vi "Main.vi"() -> ()   [LabVIEW 2016]
doc: "This Continuous Measurement sample project is based on the Queued Message Handler template.\n\nThe Event Handling Loop generates messages based on user interface actions.\n\nThe Message Handling Loop processes messages generated by the Event Handling Loop, or by other messages. There are also Acquisition and Logging message handling loop subVIs, and a chart updating loop."
uses:
  controls/UI State.ctl
  <vilib>/Analysis/baseanly.llb/Mean (DBL).vi
  <vilib>/express/express analysis/Spectral/Block/exnSpectralBlock spectral measurements PSD poly.vi
  <vilib>/express/express analysis/Spectral/Block/exnSpectralBlock spectral measurements PSD DDT.vi
  support/Message Queue/Enqueue Message (Single).vi
  <vilib>/Utility/error.llb/Error Cluster From Error Code.vi
  <vilib>/express/express analysis/Spectral/XNode/ExpressSpectralMeasurementsBlockNode.xnode
  <vilib>/ErrorRing/Error Ring.xnode
  Acquisition/Acquisition.lvlib
  Logging/Logging.lvlib
  Settings/Settings.lvlib
  support/User Event - Stop/User Event - Stop.lvlib
  support/Message Queue/Message Queue.lvlib
  <vilib>/Analysis/NI_AALBase.lvlib
panel:
  out "Y (V)":dbl format="%#_3f"
  out "X (V)":dbl format="%#_3f"
  out "Sum (V)":dbl format="%#_3f"
  out "XY Graph":cluster{"Y":dbl[], "Y":dbl[]}[](graph)
  out "Y":dynamicdata(graph)
  in  "Stop_Log":bool
  in  "Log":bool
  in  "Exit":bool
  out "Status":string
  in  "Settings":bool
  in  "Stop_Acquire":bool
  in  "Acquire":bool
  out "X":dynamicdata(graph)
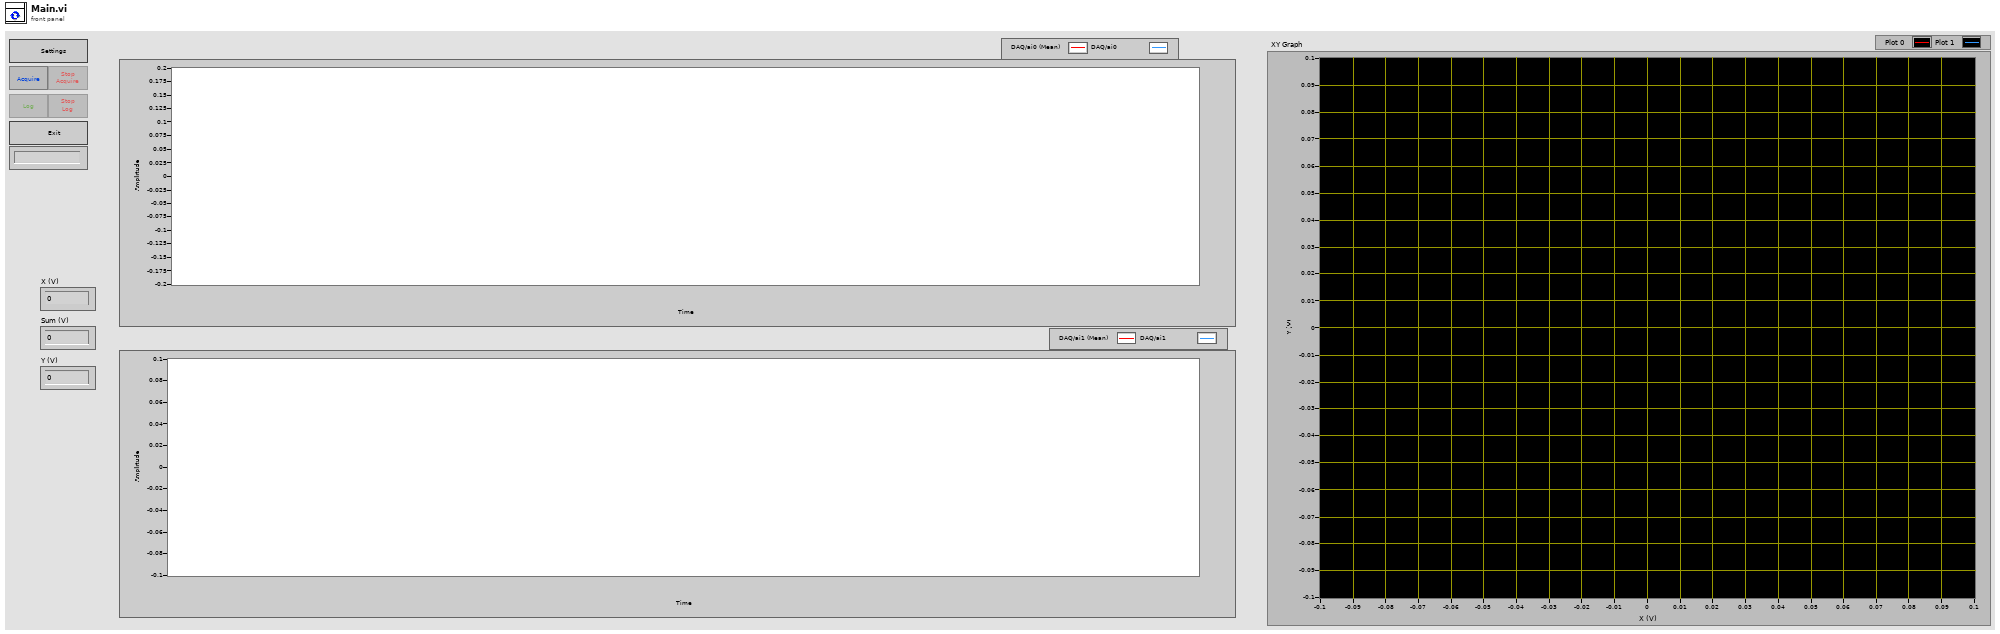
[diagram p1: front panel]
types:
  T1 = typedef "UI State.ctl" = enum16{"Idle", "Acquiring", "Acquiring Stopped", "Logging", "Logging Stopped"}
  T2 = cluster{"Acquire Ref":refnum<vi>, "Log Ref":refnum<vi>, "Stop_Acquire Ref":refnum<vi>, "Settings Ref":refnum<vi>, "Status Ref":refnum<vi>, "Exit Ref":refnum<vi>, "Stop_Log Ref":refnum<vi>}
  T3 = cluster{"Hardware Configuration":cluster{"DAQmx Channel":tag, "Max Input":dbl, "Min Input":dbl, "Sample Rate":dbl, "Channel description":string}, "Logging Configuration":cluster{"Log File Base Path":path, "TDMS File Reference":refnum<k34>, "User":string, "Data description":string}}
  T4 = typedef "Message Queue.lvlib/All Message Queues.ctl" = cluster{"UI":refnum<queue>, "Acquisition":refnum<queue>, "Logging":refnum<queue>}
  T5 = typedef "Settings.lvlib/Settings.ctl" = cluster{"Hardware Configuration":cluster{"DAQmx Channel":tag, "Max Input":dbl, "Min Input":dbl, "Sample Rate":dbl, "Channel description":string}, "Logging Configuration":cluster{"Log File Base Path":path, "TDMS File Reference":refnum<k34>, "User":string, "Data description":string}}
  T6 = cluster{"DAQmx Channel":tag, "Max Input":dbl, "Min Input":dbl, "Sample Rate":dbl, "Channel description":string}
  T7 = cluster{"Log File Base Path":path, "TDMS File Reference":refnum<k34>, "User":string, "Data description":string}
  T8 = cluster{"averaging mode":u16, "weighting mode":u16, "number of averages":u32}
  T9 = cluster{"dB On (F)":bool, "unwrap phase (F)":bool, "convert to degree (F)":bool}
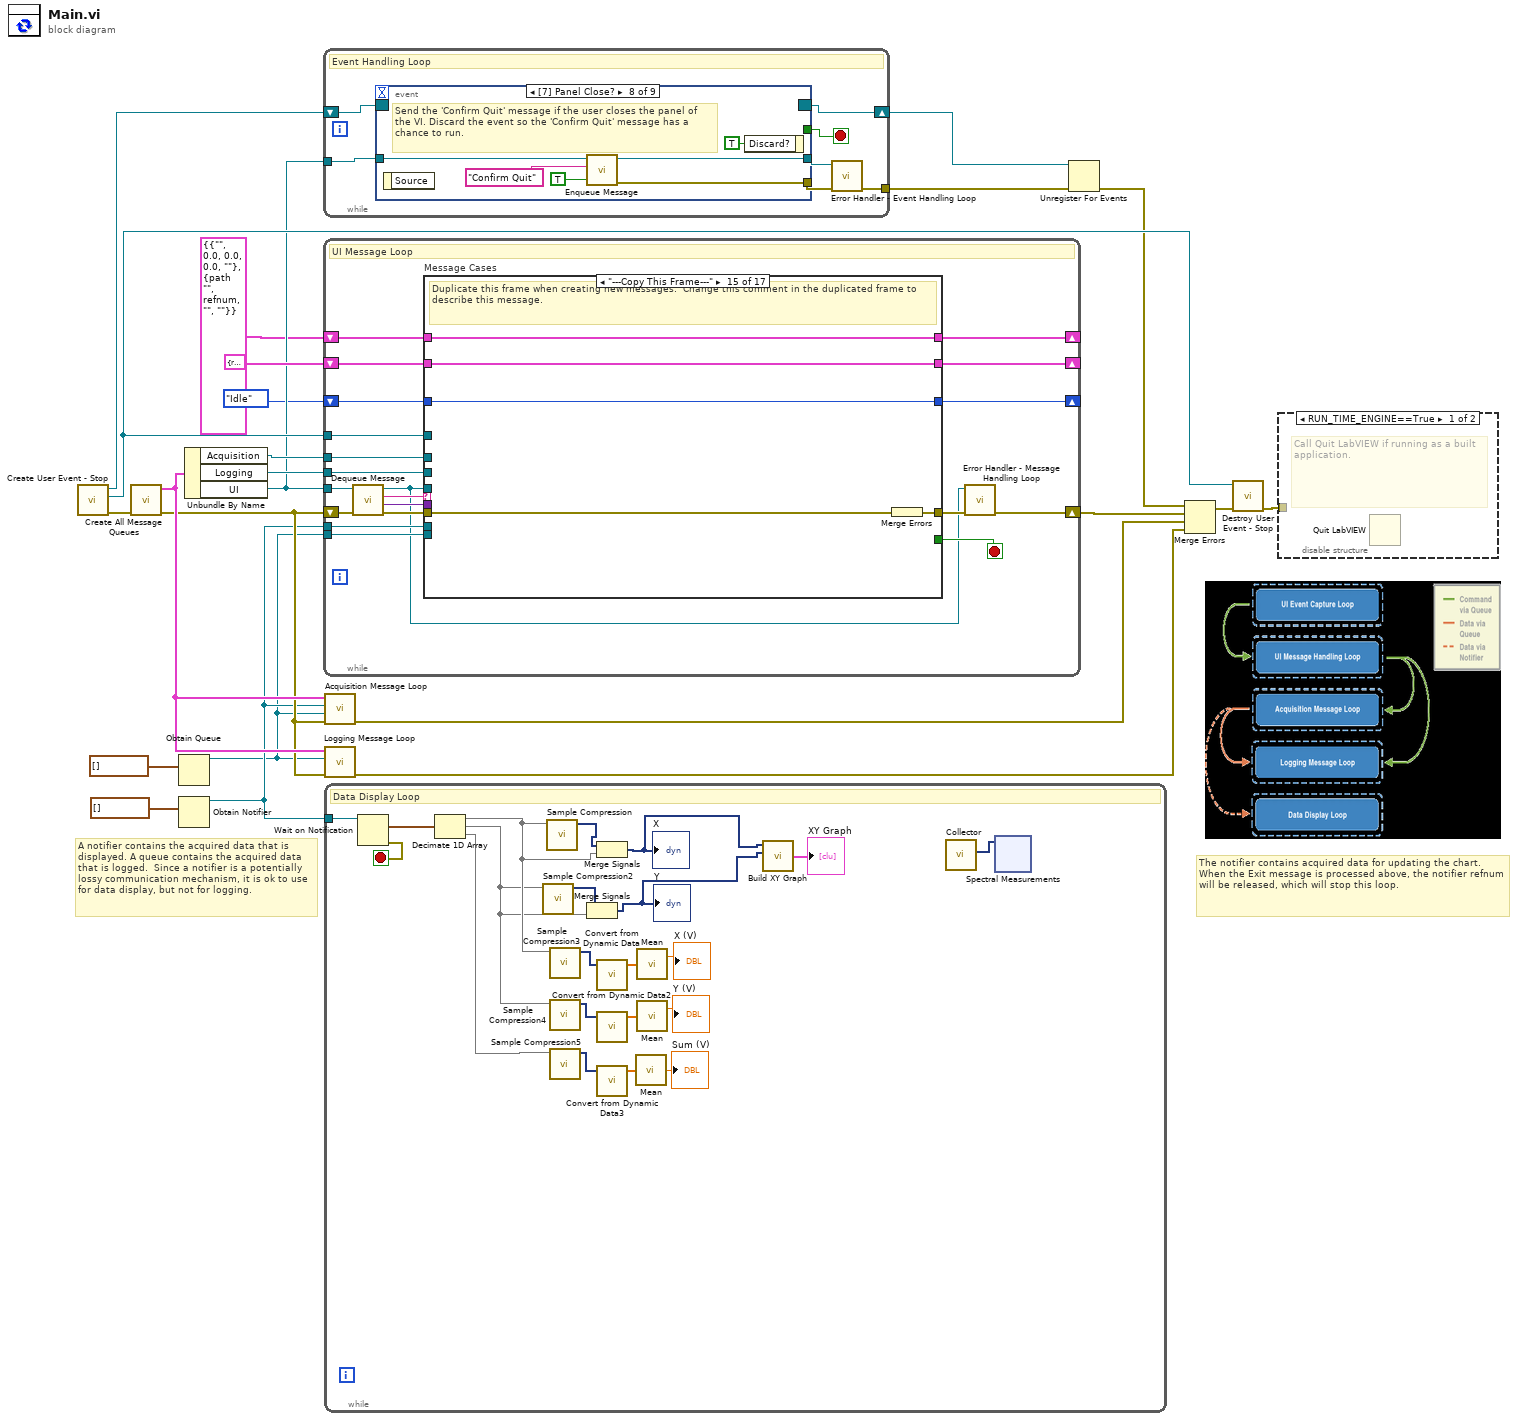
[diagram p0: block diagram]
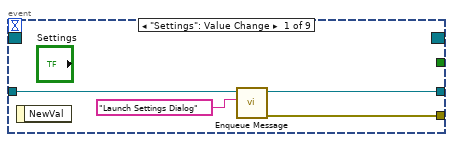
[diagram p3: hidden frame]
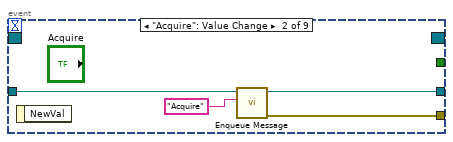
[diagram p4: hidden frame]
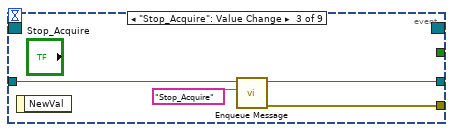
[diagram p5: hidden frame]
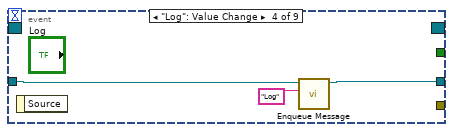
[diagram p6: hidden frame]
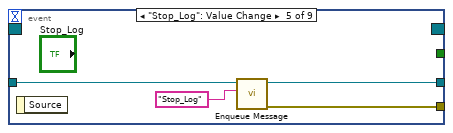
[diagram p7: hidden frame]
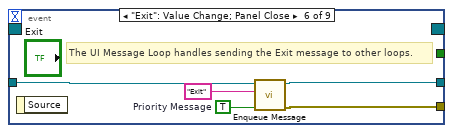
[diagram p8: hidden frame]
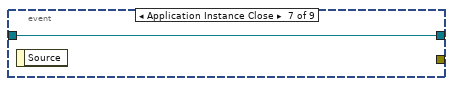
[diagram p9: hidden frame]
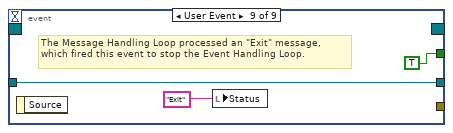
[diagram p10: hidden frame]
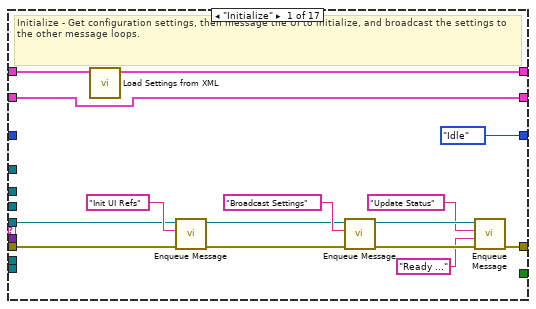
[diagram p11: hidden frame]
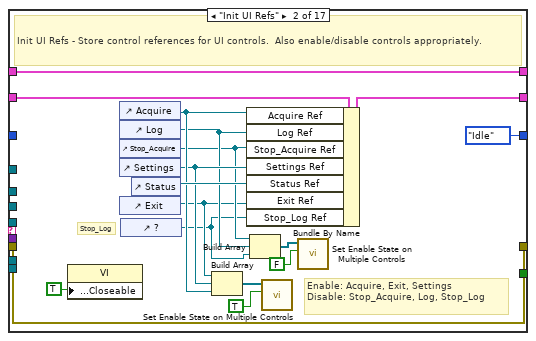
[diagram p12: hidden frame]
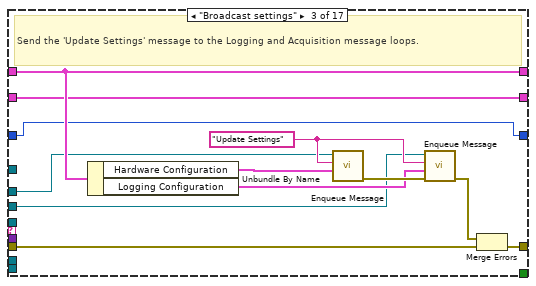
[diagram p13: hidden frame]
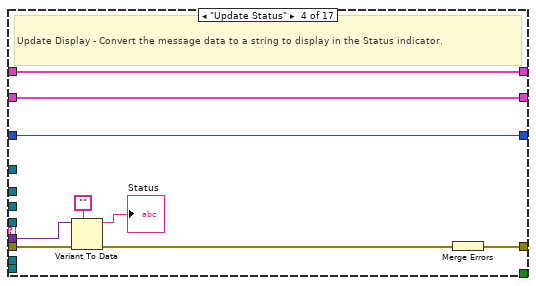
[diagram p14: hidden frame]
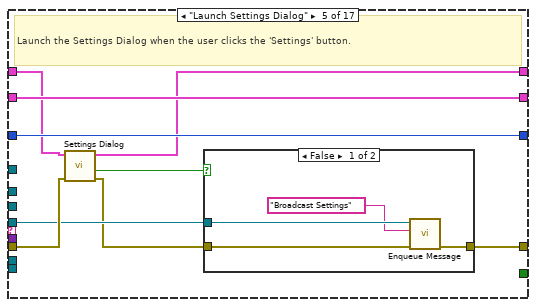
[diagram p15: hidden frame]
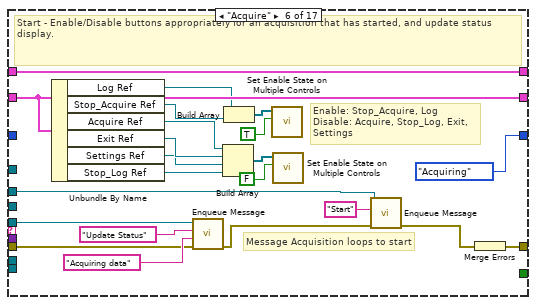
[diagram p17: hidden frame]
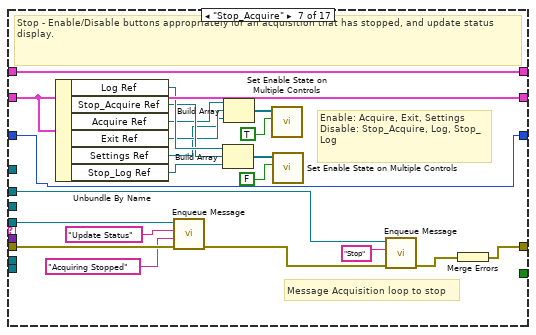
[diagram p18: hidden frame]
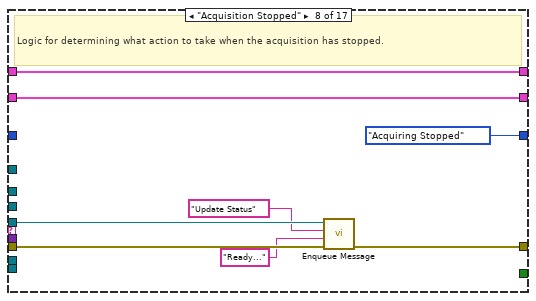
[diagram p19: hidden frame]
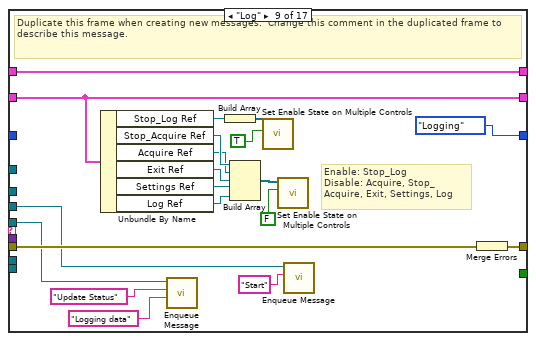
[diagram p20: hidden frame]
diagram:
  # "A notifier contains the acquired data that is displayed. A queue contains the acquired data that is logged.  Since a notifier is a potentially lossy communication mechanism, it is ok to use for data display, but not for logging."
  # "The notifier contains acquired data for updating the chart. When the Exit message is processed above, the notifier refnum will be released, which will stop this loop."
  n1 = call "Create User Event - Stop.vi"() -> ("error out"=w17:errorcluster, "User Event - Stop"=w19:refnum<user-event>, "Stop Event Registration Refnum"=w20:refnum<event-registration>)  [unwired: 9 in]
  n2 = call "Create All Message Queues.vi"("error in (no error)"=w17) -> ("error out"=w14:errorcluster, "Message Queues out"=w16:T4)  [unwired: 9 in]
  n3 = Obtain Queue(element data type=waveform(dbl)[] []) -> (queue out=w4:refnum<queue>)  [unwired: 4 in, 2 out]
  n4 = Obtain Notifier(notification data type=waveform(dbl)[] []) -> (notifier out=w6:refnum<notifier>)  [unwired: 3 in, 2 out]
  n5 = Unbundle By Name(w16) -> ("Acquisition"=w10:refnum<queue>, "Logging"=w9:refnum<queue>, "UI"=w8:refnum<queue>)
  n6 = while {
    tunnel: w8 -> [w29]
    tunnel: [w25] -> w22
    shift-right: [w28] -> w12
    shift-left: w20 -> [w30]
    stop <- w24 stop-if-true
    # "Event Handling Loop"
    n7 = event shown="[7] Panel Close?" {
      selector: w30 -> [_ _ _ _ _ _ _ _ _]
      dyn-events: [_ _ _ _ _ _ _ _ _] -> w28
      timeout: _ -> [_ _ _ _ _ _ _ _ _]
      tunnel: [_ _ _ _ _ _ _ _ TRUE ("Discard?")] -> w24
      tunnel: w29 -> [w32 w36 w41 w45 w48 w51 w55 w61 w62]
      tunnel: [w34 w38 w40 _ w47 w54 _ w56 _] -> w26
      tunnel: [w31 w35 w39 w44 w46 w50 w55 w57 w62] -> w27
      event "Settings": Value Change {
        n8 = event-data() -> ()  [unwired: 1 in, 1 out]
        n9 = call-poly "Enqueue Message.vi"("Message"="Launch Settings Dialog", "Message Queue"=w32) -> ("error out"=w34:errorcluster, "dup Message Queue"=w31:refnum<queue>)  [unwired: 8 in]
      }
      event "Acquire": Value Change {
        n10 = event-data() -> ()  [unwired: 1 in, 1 out]
        n11 = call-poly "Enqueue Message.vi"("Message"="Acquire", "Message Queue"=w36) -> ("error out"=w38:errorcluster, "dup Message Queue"=w35:refnum<queue>)  [unwired: 8 in]
      }
      event "Stop_Acquire": Value Change {
        n12 = event-data() -> ()  [unwired: 1 in, 1 out]
        n13 = call-poly "Enqueue Message.vi"("Message"="Stop_Acquire", "Message Queue"=w41) -> ("error out"=w40:errorcluster, "dup Message Queue"=w39:refnum<queue>)  [unwired: 8 in]
      }
      event "Log": Value Change {
        n14 = event-data() -> ()  [unwired: 1 in, 1 out]
        n15 = call-poly "Enqueue Message.vi"("Message"="Log", "Message Queue"=w45) -> ("dup Message Queue"=w44:refnum<queue>)  [unwired: 8 in, 1 out]
      }
      event "Stop_Log": Value Change {
        n16 = event-data() -> ()  [unwired: 1 in, 1 out]
        n17 = call-poly "Enqueue Message.vi"("Message"="Stop_Log", "Message Queue"=w48) -> ("error out"=w47:errorcluster, "dup Message Queue"=w46:refnum<queue>)  [unwired: 8 in]
      }
      event "Exit": Value Change; Panel Close {
        w52 = TRUE  # Priority Message
        # "The UI Message Loop handles sending the Exit message to other loops."
        n18 = event-data() -> ()  [unwired: 1 in, 1 out]
        n19 = call-poly "Enqueue Message.vi"("Priority Message? (F)"=w52, "Message"="Exit", "Message Queue"=w51) -> ("error out"=w54:errorcluster, "dup Message Queue"=w50:refnum<queue>)  [unwired: 7 in]
      }
      event Application Instance Close {
        n20 = event-data() -> ()  [unwired: 1 in, 1 out]
      }
      event Panel Close? {
        # "Send the 'Confirm Quit' message if the user closes the panel of the VI. Discard the event so the 'Confirm Quit' message has a chance to run."
        n21 = event-data() -> ()  [unwired: 1 in, 1 out]
        n22 = call-poly "Enqueue Message.vi"("Priority Message? (F)"=TRUE, "Message"="Confirm Quit", "Message Queue"=w61) -> ("error out"=w56:errorcluster, "dup Message Queue"=w57:refnum<queue>)  [unwired: 7 in]
        n23 = event-data("Discard?"=TRUE) -> ()  [unwired: 1 in, 1 out]
      }
      event User Event {
        # "The Message Handling Loop processed an \"Exit\" message, which fired this event to stop the Event Handling Loop."
        n24 = event-data() -> ()  [unwired: 1 in, 1 out]
        n25 = local write "Status"("Exit" ("Exit String")) -> ()
      }
    }
    n26 = call "Error Handler - Event Handling Loop.vi"("error in (no error)"=w26, "Message Queue"=w27) -> ("dup error in"=w25:errorcluster)  [unwired: 8 in, 1 out]
  }
  n27 = while {
    tunnel: w8 -> [w78]
    tunnel: w19 -> [w83]
    shift-right: [w69] -> w23
    shift-left: w14 -> [w82]
    shift-right: [w65] -> _
    shift-left: T3 {"Hardware Configuration"={"DAQmx Channel"="", "Max Input"=0.0, "Min Input"=0.0, "Sample Rate"=0.0, "Channel description"=""}, "Logging Configuration"={"Log File Base Path"=path "", "TDMS File Reference"=refnum, "User"="", "Data description"=""}} ("Settings") -> [w77]
    shift-right: [w75] -> _
    shift-left: T2 {"Acquire Ref"=refnum, "Log Ref"=refnum, "Stop_Acquire Ref"=refnum, "Settings Ref"=refnum, "Status Ref"=refnum, "Exit Ref"=refnum, "Stop_Log Ref"=refnum} ("Measurement UI Controls") -> [w76]
    tunnel: w10 -> [w74]
    tunnel: w9 -> [w73]
    tunnel: w6 -> [w72]
    tunnel: w4 -> [w71]
    shift-right: [w66] -> _
    shift-left: UI_State."Idle" ("UI State") -> [w67]
    stop <- w84 stop-if-true
    # "UI Message Loop"
    n28 = call "Dequeue Message.vi"("error in (no error)"=w82, "Message Queue"=w78) -> ("error out"=w81:errorcluster, "Message Data"=w79:variant, "Message"=w80:string, "dup Message Queue"=w68:refnum<queue>)  [unwired: 6 in]
    n29 = case "Message Cases" shown="\"---Copy This Frame---\"" w80 {
      selector: w80 -> [_ _ _ _ _ _ _ _ _ _ _ _ _ _ _ _ w334]
      tunnel: w68 -> [w89 _ _ _ w144 w172 w194 w198 w220 _ w244 w256 w272 w316 _ _ _]
      tunnel: w81 -> [w88 w116 w122 w136 w146 w152 w193 w200 w223 w240 w241 w264 w269 w320 w327 w332 _]
      tunnel: [w95 w116 w128 w137 w142 w173 w195 w199 w222 w239 w241 w265 w268 w311 w326 w331 w335] -> w70
      tunnel: [_ _ _ _ _ _ _ _ _ _ _ TRUE _ _ _ _ _] -> w84
      tunnel: w79 -> [_ _ _ w135 _ _ _ _ _ _ _ _ _ w319 _ _ _]
      tunnel: w83 -> [_ _ _ _ _ _ _ _ _ _ _ w263 _ _ _ _ _]
      tunnel: [w98 w115 w126 w132 w138 w171 w192 w203 w221 w238 w247 w261 w276 w322 w325 w330 w337] -> w65
      tunnel: w77 -> [w99 w115 w126 w132 w139 w171 w192 w203 w221 w238 w247 w261 w276 w322 w325 w330 w337]
      tunnel: w76 -> [w91 w114 w120 w131 w141 w168 w189 w202 w217 w237 w246 w259 w275 w321 w324 w329 w336]
      tunnel: [w91 w113 w120 w131 w141 w168 w189 w202 w217 w237 w246 w259 w275 w321 w324 w329 w336] -> w75
      tunnel: w74 -> [_ _ w119 _ _ w159 w185 _ _ _ _ w258 w271 _ _ _ _]
      tunnel: w73 -> [_ _ w118 _ _ _ _ _ w214 w234 _ w257 w270 _ _ _ _]
      tunnel: w72 -> [_ _ _ _ _ _ _ _ _ _ _ w255 _ _ _ _ _]
      tunnel: w71 -> [_ _ _ _ _ _ _ _ _ _ _ w251 _ _ _ _ _]
      tunnel: w67 -> [_ _ w117 w129 w140 _ w174 _ _ _ _ _ w274 w310 w323 w328 w333]
      tunnel: [UI_State."Idle" ("UI State") UI_State."Idle" ("UI State") w117 w129 w140 UI_State."Acquiring" ("UI State") w174 UI_State."Acquiring Stopped" ("UI State") UI_State."Logging" ("UI State") UI_State."Logging Stopped" ("UI State") UI_State."Logging Stopped" ("UI State") UI_State."Idle" ("UI State") w273 w310 w323 w328 w333] -> w66
      frame "Initialize" {
        # "Initialize - Get configuration settings, then message the UI to initialize, and broadcast the settings to the other message loops."
        n30 = call "Load Settings from XML.vi"("Settings in"=w99) -> ("Settings out"=w98:T5)  [unwired: 9 in, 1 out]
        n31 = call-poly "Enqueue Message.vi"("error in (no error)"=w88, "Message"="Init UI Refs", "Message Queue"=w89) -> ("error out"=w86:errorcluster, "dup Message Queue"=w87:refnum<queue>)  [unwired: 7 in]
        n32 = call-poly "Enqueue Message.vi"("error in (no error)"=w86, "Message"="Broadcast Settings", "Message Queue"=w87) -> ("error out"=w97:errorcluster, "dup Message Queue"=w96:refnum<queue>)  [unwired: 7 in]
        n33 = call-poly "Enqueue Message.vi"("error in (no error)"=w97, "Message Data"="Ready ..." ("Ready..."), "Message"="Update Status", "Message Queue"=w96) -> ("error out"=w95:errorcluster)  [unwired: 6 in, 1 out]
      }
      frame "Init UI Refs" {
        # "Stop_Log"
        # "Enable: Acquire, Exit, Settings\nDisable: Stop_Acquire, Log, Stop_Log"
        # "Init UI Refs - Store control references for UI controls.  Also enable/disable controls appropriately."
        n34 = property class="VI"("Front Panel.Closeable"=TRUE ("Front Panel Window:Closeable")) -> ()  [unwired: 2 in, 2 out]
        n35 = control-ref of="Acquire"() -> (w109:refnum<vi>)
        n36 = control-ref of="Log"() -> (w105:refnum<vi>)
        n37 = control-ref of="Stop_Acquire"() -> (w104:refnum<vi>)
        n38 = control-ref of="Settings"() -> (w106:refnum<vi>)
        n39 = control-ref of="Exit"() -> (w101:refnum<vi>)
        n40 = control-ref of="?"() -> (w100:refnum<vi>)
        n41 = control-ref of="Status"() -> (w110:refnum<vi>)
        n42 = Build Array(w101, w106, w109) -> (w108:refnum<vi>[])
        n43 = Bundle By Name(cluster=w114, "Acquire Ref"=w109, "Log Ref"=w105, "Stop_Acquire Ref"=w104, "Settings Ref"=w106, "Status Ref"=w110, "Exit Ref"=w101, "Stop_Log Ref"=w100) -> (w113:T2)
        n44 = Build Array(w104, w105, w100) -> (w103:refnum<vi>[])
        n45 = call "Set Enable State on Multiple Controls.vi"("Enable?"=TRUE, "Controls"=w108) -> ()  [unwired: 10 in]
        n46 = call "Set Enable State on Multiple Controls.vi"("Enable?"=FALSE, "Controls"=w103) -> ()  [unwired: 10 in]
      }
      frame "Broadcast settings" {
        w121 = "Update Settings" ("Message")
        # "Send the 'Update Settings' message to the Logging and Acquisition message loops."
        n47 = Unbundle By Name(w126) -> ("Hardware Configuration"=w125:T6, "Logging Configuration"=w124:T7)
        n48 = call-poly "Enqueue Message.vi"("Message Data"=w125, "Message"=w121, "Message Queue"=w119) -> ("error out"=w127:errorcluster)  [unwired: 7 in, 1 out]
        n49 = call-poly "Enqueue Message.vi"("error in (no error)"=w127, "Message Data"=w124, "Message"=w121, "Message Queue"=w118) -> ("error out"=w123:errorcluster)  [unwired: 6 in, 1 out]
        n50 = Merge Errors(w123, w122) -> (w128:errorcluster)
      }
      frame "Update Status" {
        # "Update Display - Convert the message data to a string to display in the Status indicator."
        n51 = Variant To Data(error in=w136, type="", Variant=w135) -> (data=→"Status":string, error out=w133:errorcluster)
        n52 = Merge Errors(w133) -> (w137:errorcluster)
      }
      frame "Launch Settings Dialog" {
        # "Launch the Settings Dialog when the user clicks the 'Settings' button."
        n53 = call "Settings Dialog.vi"("error in (no error)"=w146, "Settings in"=w139) -> ("error out"=w143:errorcluster, "Cancelled?"=w145:bool, "Settings out"=w138:T3)  [unwired: 6 in, 1 out]
        n54 = case shown="False" w145 {
          tunnel: w144 -> [w150 _]
          tunnel: w143 -> [w149 w151]
          tunnel: [w148 w151] -> w142
          frame False {
            n55 = call-poly "Enqueue Message.vi"("error in (no error)"=w149, "Message"="Broadcast Settings", "Message Queue"=w150) -> ("error out"=w148:errorcluster)  [unwired: 7 in, 1 out]
          }
          frame True {
          }
        }
      }
      frame "Acquire" {
        # "Message Acquisition loops to start"
        # "Enable: Stop_Acquire, Log\nDisable: Acquire, Stop_Log, Exit, Settings"
        # "Start - Enable/Disable buttons appropriately for an acquisition that has started, and update status display."
        n56 = Unbundle By Name(w168) -> ("Log Ref"=w156:refnum<vi>, "Stop_Acquire Ref"=w157:refnum<vi>, "Acquire Ref"=w163:refnum<vi>, "Exit Ref"=w162:refnum<vi>, "Settings Ref"=w161:refnum<vi>, "Stop_Log Ref"=w153:refnum<vi>)
        n57 = call-poly "Enqueue Message.vi"("error in (no error)"=w152, "Message Data"="Acquiring data" ("Waiting for trigger"), "Message"="Update Status", "Message Queue"=w172) -> ("error out"=w154:errorcluster)  [unwired: 6 in, 1 out]
        n58 = Build Array(w163, w162, w161, w153) -> (w166:refnum<vi>[])
        n59 = Build Array(w156, w157) -> (w165:refnum<vi>[])
        n60 = call "Set Enable State on Multiple Controls.vi"("Enable?"=TRUE, "Controls"=w165) -> ()  [unwired: 10 in]
        n61 = call "Set Enable State on Multiple Controls.vi"("Enable?"=FALSE, "Controls"=w166) -> ()  [unwired: 10 in]
        n62 = call-poly "Enqueue Message.vi"("error in (no error)"=w154, "Message"="Start", "Message Queue"=w159) -> ("error out"=w160:errorcluster)  [unwired: 7 in, 1 out]
        n63 = Merge Errors(w160) -> (w173:errorcluster)
      }
      frame "Stop_Acquire" {
        # "Message Acquisition loop to stop"
        # "Enable: Acquire, Exit, Settings\nDisable: Stop_Acquire, Log, Stop_Log"
        # "Stop - Enable/Disable buttons appropriately for an acquisition that has stopped, and update status display."
        n64 = Unbundle By Name(w189) -> ("Log Ref"=w183:refnum<vi>, "Stop_Acquire Ref"=w182:refnum<vi>, "Acquire Ref"=w181:refnum<vi>, "Exit Ref"=w180:refnum<vi>, "Settings Ref"=w179:refnum<vi>, "Stop_Log Ref"=w178:refnum<vi>)
        n65 = call-poly "Enqueue Message.vi"("error in (no error)"=w193, "Message Data"="Acquiring Stopped" ("Ready..."), "Message"="Update Status", "Message Queue"=w194) -> ("error out"=w177:errorcluster)  [unwired: 6 in, 1 out]
        n66 = Build Array(w183, w182, w178) -> (w175:refnum<vi>[])
        n67 = Build Array(w181, w180, w179) -> (w176:refnum<vi>[])
        n68 = call "Set Enable State on Multiple Controls.vi"("Enable?"=TRUE, "Controls"=w176) -> ()  [unwired: 10 in]
        n69 = call "Set Enable State on Multiple Controls.vi"("Enable?"=FALSE, "Controls"=w175) -> ()  [unwired: 10 in]
        n70 = call-poly "Enqueue Message.vi"("error in (no error)"=w177, "Message"="Stop", "Message Queue"=w185) -> ("error out"=w186:errorcluster)  [unwired: 7 in, 1 out]
        n71 = Merge Errors(w186) -> (w195:errorcluster)
      }
      frame "Acquisition Stopped" {
        # "Logic for determining what action to take when the acquisition has stopped."
        n72 = call-poly "Enqueue Message.vi"("error in (no error)"=w200, "Message Data"="Ready..." ("Message"), "Message"="Update Status", "Message Queue"=w198) -> ("error out"=w199:errorcluster)  [unwired: 6 in, 1 out]
      }
      frame "Log" {
        # "Enable: Stop_Log\nDisable: Acquire, Stop_Acquire, Exit, Settings, Log"
        # "Duplicate this frame when creating new messages.  Change this comment in the duplicated frame to describe this message."
        n73 = Unbundle By Name(w217) -> ("Stop_Log Ref"=w212:refnum<vi>, "Stop_Acquire Ref"=w210:refnum<vi>, "Acquire Ref"=w209:refnum<vi>, "Exit Ref"=w208:refnum<vi>, "Settings Ref"=w207:refnum<vi>, "Log Ref"=w206:refnum<vi>)
        n74 = call-poly "Enqueue Message.vi"("Message Data"="Logging data" ("Ready..."), "Message"="Update Status", "Message Queue"=w220) -> ()  [unwired: 7 in, 2 out]
        n75 = Build Array(w212) -> (w211:refnum<vi>[])
        n76 = Build Array(w210, w209, w208, w207, w206) -> (w205:refnum<vi>[])
        n77 = call "Set Enable State on Multiple Controls.vi"("Enable?"=TRUE, "Controls"=w211) -> ()  [unwired: 10 in]
        n78 = call "Set Enable State on Multiple Controls.vi"("Enable?"=FALSE, "Controls"=w205) -> ()  [unwired: 10 in]
        n79 = call-poly "Enqueue Message.vi"("Message"="Start", "Message Queue"=w214) -> ()  [unwired: 8 in, 2 out]
        n80 = Merge Errors(w223) -> (w222:errorcluster)
      }
      frame "Stop_Log" {
        # "Message Logging loop to stop"
        # "Enable: Log, Stop_Acquire\nDisable: Acquire, Exit, Settings, Stop_Log"
        # "Duplicate this frame when creating new messages.  Change this comment in the duplicated frame to describe this message."
        n81 = Unbundle By Name(w237) -> ("Stop_Acquire Ref"=w232:refnum<vi>, "Log Ref"=w226:refnum<vi>, "Acquire Ref"=w230:refnum<vi>, "Exit Ref"=w229:refnum<vi>, "Settings Ref"=w228:refnum<vi>, "Stop_Log Ref"=w225:refnum<vi>)
        n82 = Build Array(w232, w226) -> (w231:refnum<vi>[])
        n83 = Build Array(w225, w230, w229, w228) -> (w227:refnum<vi>[])
        n84 = call "Set Enable State on Multiple Controls.vi"("Enable?"=TRUE, "Controls"=w231) -> ()  [unwired: 10 in]
        n85 = call "Set Enable State on Multiple Controls.vi"("Enable?"=FALSE, "Controls"=w227) -> ()  [unwired: 10 in]
        n86 = call-poly "Enqueue Message.vi"("Message"="Stop", "Message Queue"=w234) -> ()  [unwired: 8 in, 2 out]
        n87 = Merge Errors(w240) -> (w239:errorcluster)
      }
      frame "Logging Stopped" {
        # "Logic for determining what action to take when the logging has stopped."
        n88 = call-poly "Enqueue Message.vi"("Message Data"="Acquiring data" ("Ready..."), "Message"="Update Status", "Message Queue"=w244) -> ()  [unwired: 7 in, 2 out]
      }
      frame "Exit" {
        w260 = "Exit" ("Message")
        # "Don't check the error outs. The acquisition and logging queues may have already been released."
        # "Close references owned by the Main VI."
        # "Stop the VI"
        # "Exit - Fire the User Event to stop the Event Handling Loop.  Also send Exit messages to the Acquisition and Logging loops."
        n89 = Release Queue(queue=w256, error in (no error)=w264) -> (error out=w254:errorcluster)  [unwired: 1 in, 2 out]
        n90 = call "Fire User Event - Stop.vi"("User Event - Stop"=w263) -> ("error out"=w262:errorcluster)  [unwired: 10 in]
        n91 = Release Notifier(notifier=w255, error in (no error)=w254) -> (error out=w253:errorcluster)  [unwired: 1 in, 2 out]
        n92 = Release Queue(queue=w251, error in (no error)=w253) -> (error out=w252:errorcluster)  [unwired: 1 in, 2 out]
        n93 = call-poly "Enqueue Message.vi"("Priority Message? (F)"=TRUE, "Message"=w260, "Message Queue"=w258) -> ()  [unwired: 7 in, 2 out]
        n94 = call-poly "Enqueue Message.vi"("Priority Message? (F)"=TRUE, "Message"=w260, "Message Queue"=w257) -> ()  [unwired: 7 in, 2 out]
        n95 = Merge Errors(w262, w252) -> (w265:errorcluster)
      }
      frame "Confirm Quit" {
        # "Confirm Quit - Message that can confirm whether or not the user wants to exit the application."
        n96 = case shown="\"Idle\", Default" w274 {
          tunnel: [w279 w284 w290 w295 w303] -> w267
          tunnel: [UI_State."Idle" ("UI State") UI_State."Acquiring" ("UI State") UI_State."Idle" ("UI State") UI_State."Logging" ("UI State") UI_State."Acquiring" ("UI State")] -> w273
          tunnel: w272 -> [w277 w283 w293 w298 w305]
          tunnel: w271 -> [_ w286 _ _ w308]
          tunnel: w269 -> [_ _ _ _ _]
          tunnel: w270 -> [_ _ _ w301 _]
          frame "Idle", Default {
            # "If 'Confirm Quit' comes in while the system is idle, there is no need for a confirmation message."
            n97 = call-poly "Enqueue Message.vi"("Priority Message? (F)"=TRUE, "Message"="Exit", "Message Queue"=w277) -> ("error out"=w279:errorcluster)  [unwired: 7 in, 1 out]
          }
          frame "Acquiring" {
            n98 = call-poly "Enqueue Message.vi"("Priority Message? (F)"=TRUE, "Message"="Stop", "Message Queue"=w286) -> ("error out"=w285:errorcluster)  [unwired: 7 in, 1 out]
            n99 = call-poly "Enqueue Message.vi"("error in (no error)"=w285, "Message"="Confirm Quit", "Message Queue"=w283) -> ("error out"=w284:errorcluster)  [unwired: 7 in, 1 out]
          }
          frame "Acquiring Stopped" {
            n100 = call-poly "Enqueue Message.vi"("Priority Message? (F)"=TRUE, "Message"="Exit", "Message Queue"=w293) -> ("error out"=w290:errorcluster)  [unwired: 7 in, 1 out]
          }
          frame "Logging" {
            n101 = call-poly "Enqueue Message.vi"("Priority Message? (F)"=TRUE, "Message"="Stop", "Message Queue"=w301) -> ("error out"=w296:errorcluster)  [unwired: 7 in, 1 out]
            n102 = call-poly "Enqueue Message.vi"("error in (no error)"=w296, "Message"="Confirm Quit", "Message Queue"=w298) -> ("error out"=w295:errorcluster)  [unwired: 7 in, 1 out]
          }
          frame "Logging Stopped" {
            n103 = call-poly "Enqueue Message.vi"("Priority Message? (F)"=TRUE, "Message"="Stop", "Message Queue"=w308) -> ()  [unwired: 7 in, 2 out]
            n104 = call-poly "Enqueue Message.vi"("Message"="Confirm Quit", "Message Queue"=w305) -> ("error out"=w303:errorcluster)  [unwired: 8 in, 1 out]
          }
        }
        n105 = Merge Errors(w267, w269) -> (w268:errorcluster)
      }
      frame "Error" {
        # "Error - Check the error message data and respond accordingly. This message is sent by the \"Error Handler\" VIs at the end of each loop in this application."
        n106 = Variant To Data(error in=w320, type=errorcluster {"status"=FALSE, "code"=0, "source"=""} ("error out"), Variant=w319) -> (data=w317:errorcluster, error out=w313:errorcluster)
        n107 = call <vilib>:"Simple Error Handler.vi"("error in (no error)"=w317) -> ()  [unwired: 4 in, 5 out]
        n108 = call-poly "Enqueue Message.vi"("Priority Message? (F)"=TRUE, "Message"="Exit", "Message Queue"=w316) -> ("error out"=w312:errorcluster)  [unwired: 7 in, 1 out]
        n109 = Merge Errors(w312, w313) -> (w311:errorcluster)
      }
      frame "---Copy This Frame---" {
        # "Duplicate this frame when creating new messages.  Change this comment in the duplicated frame to describe this message."
        n110 = Merge Errors(w327) -> (w326:errorcluster)
      }
      frame " Display Setting" {
        # "Duplicate this frame when creating new messages.  Change this comment in the duplicated frame to describe this message."
        n111 = Merge Errors(w332) -> (w331:errorcluster)
      }
      frame Default {
        # "'Default' case only runs if there is a message that isn't defined in any of the other cases.  Output a programming error."
        n112 = xnode "Error Ring"("parameter 0"=w334) -> ("error out"=w335:errorcluster)
      }
    }
    n113 = call "Error Handler - Message Handling Loop.vi"("error in (no error)"=w70, "Message Queue"=w68) -> ("dup error in"=w69:errorcluster)  [unwired: 8 in, 1 out]
  }
  n114 = call "Acquisition Message Loop.vi"("error in (no error)"=w14, "Data Queue"=w4, "Data Notifier"=w6, "Message Queues"=w16) -> ("error out"=w18:errorcluster)  [unwired: 7 in]
  n115 = call "Logging Message Loop.vi"("error in (no error)"=w14, "Data Queue"=w4, "Message Queues"=w16) -> ("error out"=w15:errorcluster)  [unwired: 8 in]
  n116 = while "Data Display Loop" {
    tunnel: w6 -> [w365]
    stop <- w361 stop-if-true
    # "Data Display Loop"
    n117 = Wait on Notification(notifier=w365) -> (notification=w363:waveform(dbl)[], error out=w361:errorcluster)  [unwired: 3 in, 2 out]
    n118 = Decimate 1D Array(w363) -> (w348:waveform(dbl)[], w347:waveform(dbl)[], w351:waveform(dbl)[])
    n119 = call "Sample Compression2"("Signals"=w347) -> ("Mean"=w356:dynamicdata)  [unwired: 8 in, 2 out]
    n120 = call "Sample Compression"("Signals"=w348) -> ("Mean"=w357:dynamicdata)  [unwired: 8 in, 2 out]
    n121 = call "Sample Compression3"("Signals"=w348) -> ("Mean"=w355:dynamicdata)  [unwired: 8 in, 2 out]
    n122 = call "Sample Compression4"("Signals"=w347) -> ("Mean"=w353:dynamicdata)  [unwired: 8 in, 2 out]
    n123 = call "Sample Compression5"("Signals"=w351) -> ("Mean"=w350:dynamicdata)  [unwired: 8 in, 2 out]
    n124 = Merge Signals(w356, w347) -> (w345:dynamicdata)
    "Y" <- w345
    n125 = Merge Signals(w357, w348) -> (w346:dynamicdata)
    "X" <- w346
    n126 = call "Convert from Dynamic Data"("Dynamic Data Type"=w355) -> ("Array"=w354:dbl[])  [unwired: 3 in]
    n127 = call "Convert from Dynamic Data2"("Dynamic Data Type"=w353) -> ("Array"=w352:dbl[])  [unwired: 3 in]
    n128 = call "Convert from Dynamic Data3"("Dynamic Data Type"=w350) -> ("Array"=w349:dbl[])  [unwired: 3 in]
    n129 = call-poly <vilib>:"Mean.vi"("X"=w349) -> ("mean"=→"Sum (V)":dbl)  [unwired: 1 out]
    n130 = call-poly <vilib>:"Mean.vi"("X"=w354) -> ("mean"=→"X (V)":dbl)  [unwired: 1 out]
    n131 = call-poly <vilib>:"Mean.vi"("X"=w352) -> ("mean"=→"Y (V)":dbl)  [unwired: 1 out]
    n132 = call "Build XY Graph"("Y Input"=w345, "X Input"=w346) -> ("XY Graph"=→"XY Graph":cluster{"Y":dbl[], "Y":dbl[]}[])  [unwired: 3 in, 6 out]
    n133 = call "Collector"() -> ("Collected Signals"=w364:dynamicdata)  [unwired: 10 in, 1 out]
    n134 = xnode "Spectral Measurements"("Signals"=w364) -> ()  [unwired: 1 in, 2 out]
  }
  n135 = Unregister For Events(event registration refnum=w12, error in=w22) -> (error out=w13:errorcluster)
  n136 = Merge Errors(w13, w23, w18, w15) -> (w21:errorcluster)
  n137 = call "Destroy User Event - Stop.vi"("error in (no error)"=w21, "User Event - Stop"=w19) -> ("error out"=w3:errorcluster)  [unwired: 9 in]
  n138 = disable-structure shown="RUN_TIME_ENGINE==True" {
    disable-tunnel: w3 -> [_ _]
    frame condition #0 {
      # "Call Quit LabVIEW if running as a built application."
      n139 = Quit LabVIEW() -> ()  [unwired: 1 in]
    }
    frame condition #1 (active) {
    }
  }
